vi "Analysis.Data Dump, Sel Results to 1D Str.vi"(7 "ValStr":variant, 10 "Result Summary":T1, 11 "Names":string[](array[string])=["Location", "SN", "Start Time", "Result", "Result Code", "Result Desc"]) -> (3 "Data List out":string[](array[string]))   [LabVIEW 2024]
uses:
  Analysis.Result Summary_V2.ctl
  Time/Time.Format Selector.ctl
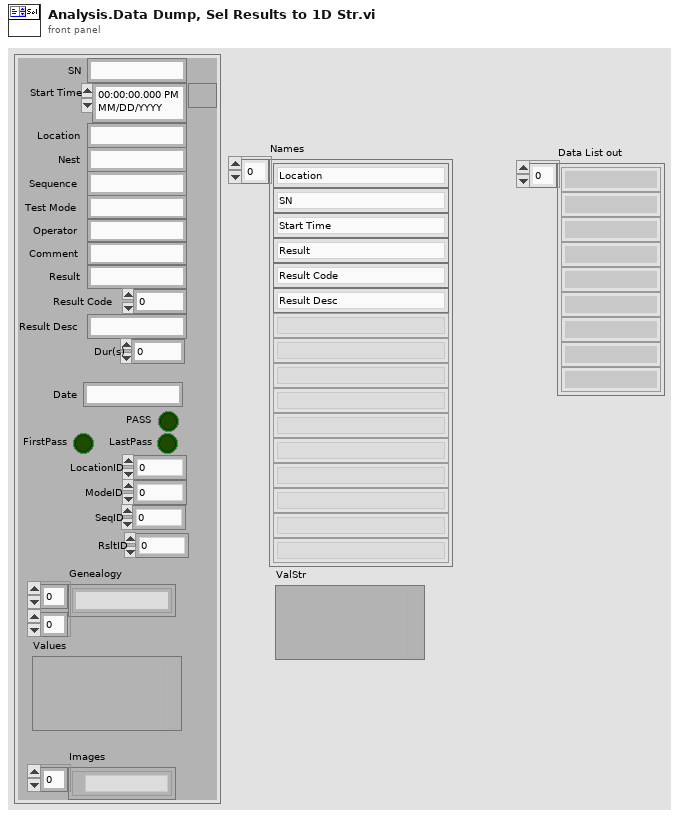
[diagram p1: front panel]
types:
  T1 = typedef "Analysis.Result Summary_V2.ctl" = cluster{"SN":string, "Start Time":timestamp, "Location":string, "Nest":string, "Sequence":string, "Operator":string, "Test Mode":string, "Comment":string, "Result":string, "Result Code":i32, "Result Desc":string, "Date":string, "Dur(s)":dbl, "PASS":bool, "FirstPass":bool, "LastPass":bool, "LocationID":i32, "ModeID":i32, "SeqID":i32, "RsltID":i32, "Genealogy":string[][], "Values":variant, "Images":path[]}
  T2 = typedef "Time.Format Selector.ctl" = enum16{"yyyy/mm/dd HH:MM:S.sss", "yyyy/mm/dd HH:MM:SS", "yyyy-MM-ddTHH:mm:ss[.mmm]", "YYYYMMDD_HHMMSS"}
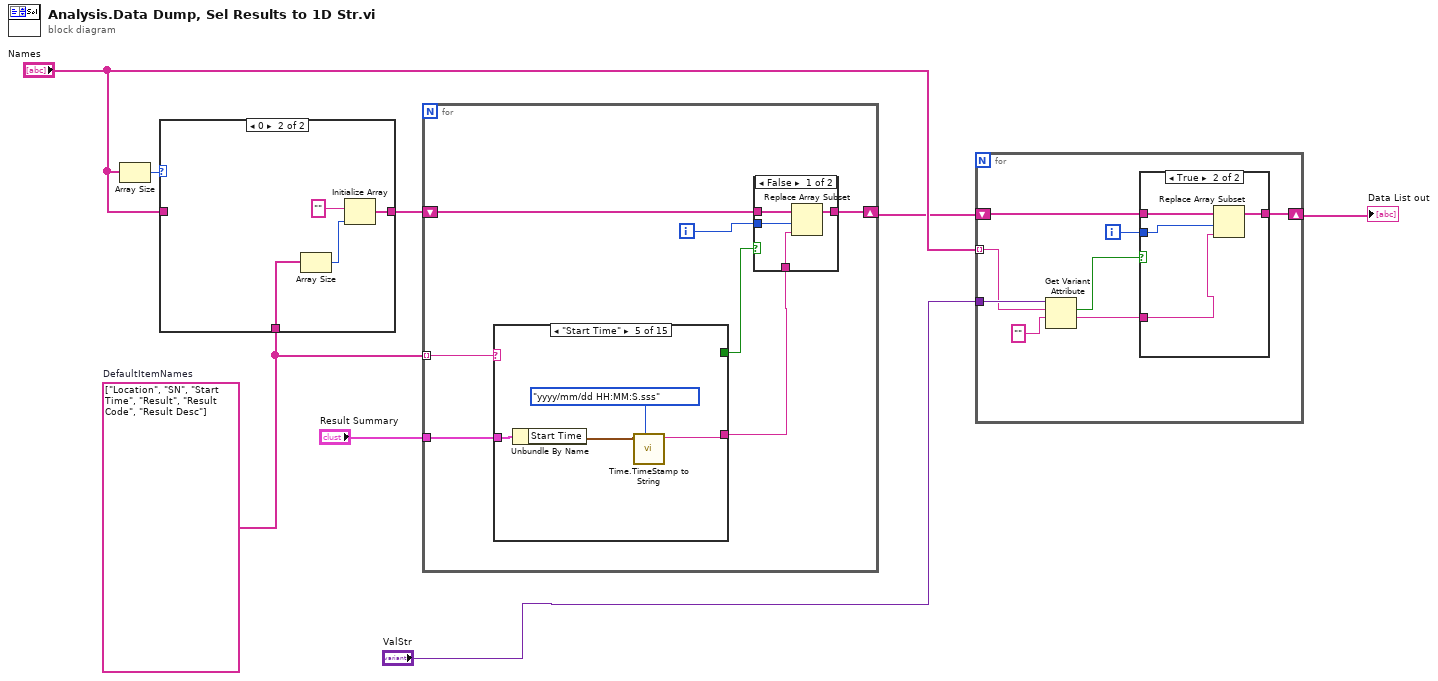
[diagram p0: block diagram]
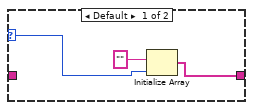
[diagram p3: hidden frame]
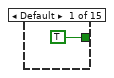
[diagram p5: hidden frame]
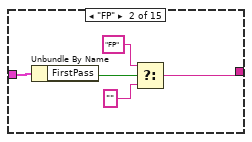
[diagram p6: hidden frame]
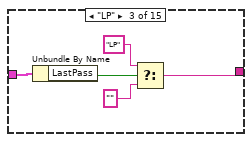
[diagram p7: hidden frame]
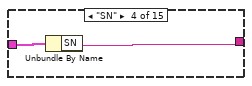
[diagram p8: hidden frame]
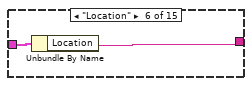
[diagram p9: hidden frame]
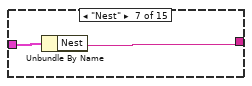
[diagram p10: hidden frame]
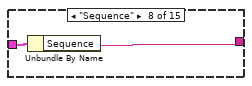
[diagram p11: hidden frame]
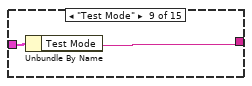
[diagram p12: hidden frame]
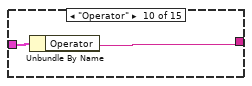
[diagram p13: hidden frame]
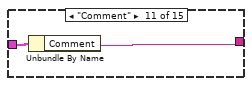
[diagram p14: hidden frame]
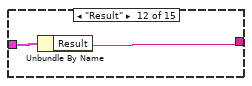
[diagram p15: hidden frame]
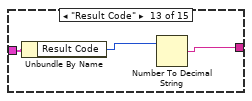
[diagram p16: hidden frame]
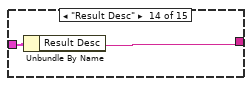
[diagram p17: hidden frame]
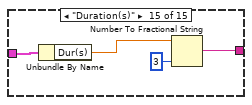
[diagram p18: hidden frame]
diagram:
  w6 = string[] ["Location", "SN", "Start Time", "Result", "Result Code", "Result Desc"]  # DefaultItemNames
  n1 = Array Size(array="Names") -> (size(s)=w8:i32)
  n2 = case shown="0" w8 {
    selector: w8 -> [w10 _]
    tunnel: [w9 w14] -> w7
    tunnel: "Names" -> [_ _]
    tunnel: w6 -> [_ w13]
    frame Default {
      n3 = Initialize Array("", w10) -> (w9:string[])
    }
    frame 0 {
      n4 = Array Size(array=w13) -> (size(s)=w12:i32)
      n5 = Initialize Array("", w12) -> (w14:string[])
    }
  }
  n6 = for {
    shift-right: [w21] -> w3
    shift-left: w7 -> [w22]
    tunnel: "Result Summary" -> [w19]
    tunnel: w6 -> [w18] mode=indexing
    i -> [w17]
    n7 = case shown="\"Start Time\"" w18 {
      tunnel: [_ w31 w36 w39 w42 w45 w47 w49 w51 w53 w55 w57 w59 w62 w64] -> w20
      tunnel: w19 -> [_ w33 w38 w40 w44 w46 w48 w50 w52 w54 w56 w58 w61 w63 w67]
      tunnel: [TRUE _ _ _ _ _ _ _ _ _ _ _ _ _ _] -> w16
      frame Default {
      }
      frame "FP" {
        n8 = Unbundle By Name(w33) -> ("FirstPass"=w32:bool)
        n9 = Select(t="FP", s=w32, f="") -> (s? t:f=w31:string)
      }
      frame "LP" {
        n10 = Unbundle By Name(w38) -> ("LastPass"=w37:bool)
        n11 = Select(t="LP", s=w37, f="") -> (s? t:f=w36:string)
      }
      frame "SN" {
        n12 = Unbundle By Name(w40) -> ("SN"=w39:string)
      }
      frame "Start Time" {
        n13 = Unbundle By Name(w44) -> ("Start Time"=w43:timestamp)
        n14 = call "Time.TimeStamp to String.vi"("TimeFormat"=Time.Format_Selector."yyyy/mm/dd HH:MM:S.sss", "Time Stamp in"=w43) -> ("Time String Out"=w42:string)  [unwired: 9 in]
      }
      frame "Location" {
        n15 = Unbundle By Name(w46) -> ("Location"=w45:string)
      }
      frame "Nest" {
        n16 = Unbundle By Name(w48) -> ("Nest"=w47:string)
      }
      frame "Sequence" {
        n17 = Unbundle By Name(w50) -> ("Sequence"=w49:string)
      }
      frame "Test Mode" {
        n18 = Unbundle By Name(w52) -> ("Test Mode"=w51:string)
      }
      frame "Operator" {
        n19 = Unbundle By Name(w54) -> ("Operator"=w53:string)
      }
      frame "Comment" {
        n20 = Unbundle By Name(w56) -> ("Comment"=w55:string)
      }
      frame "Result" {
        n21 = Unbundle By Name(w58) -> ("Result"=w57:string)
      }
      frame "Result Code" {
        n22 = Unbundle By Name(w61) -> ("Result Code"=w60:i32)
        n23 = Number To Decimal String(number=w60) -> (decimal integer string=w59:string)  [unwired: 1 in]
      }
      frame "Result Desc" {
        n24 = Unbundle By Name(w63) -> ("Result Desc"=w62:string)
      }
      frame "Duration(s)" {
        n25 = Unbundle By Name(w67) -> ("Dur(s)"=w66:dbl)
        n26 = Number To Fractional String(number=w66, precision (6)=i16 3) -> (F-format string=w64:string)  [unwired: 2 in]
      }
    }
    n27 = case shown="False" w16 {
      tunnel: w22 -> [w26 w27]
      tunnel: [w25 w27] -> w21
      tunnel: w20 -> [w24 _]
      tunnel: w17 -> [w23 _]
      frame False {
        n28 = Replace Array Subset(array=w26, new element=w24, index=w23) -> (w25:string[])
      }
      frame True {
      }
    }
  }
  n29 = for {
    tunnel: "Names" -> [w71] mode=indexing
    shift-right: [w73] -> w2
    shift-left: w3 -> [w75]
    tunnel: "ValStr" -> [w72]
    i -> [w70]
    n30 = Get Variant Attribute(Variant=w72, name=w71, default value (empty Variant)="") -> (found=w74:bool, value=w68:string)  [unwired: 1 in, 2 out]
    n31 = case shown="True" w74 {
      tunnel: w75 -> [w76 w80]
      tunnel: [w76 w79] -> w73
      tunnel: w70 -> [_ w78]
      tunnel: w68 -> [_ w77]
      frame False {
      }
      frame True {
        n32 = Replace Array Subset(array=w80, new element=w77, index=w78) -> (w79:string[])
      }
    }
  }
  "Data List out" <- w2
